vi "Cal RHS (Numeric).vi"(8 "error in (no error)":errorcluster, 10 "RHS in":variant, 11 "Domain_Steady_2D_Polygon in":refnum<class "NI_Domain_Steady_2D_Polygon.lvclass">) -> (0 "error out":errorcluster, 2 "RHS out":variant, 3 "Domain_Steady_2D_Polygon out":refnum<class "NI_Domain_Steady_2D_Polygon.lvclass">)   [LabVIEW 2017, in "NI_PDE.lvlib" / "NI_Domain_Steady_2D_Polygon.lvclass"]
uses:
  <vilib>/gmath/pde.llb/DomainClass/Domain_Steady_2D_Polygon/NI_Domain_Steady_2D_Polygon.lvclass
  <vilib>/gmath/pde.llb/DomainClass/Domain_Steady_2D_Polygon/NI_Domain_Steady_2D_Polygon.lvclass/NI_Domain_Steady_2D_Polygon.ctl
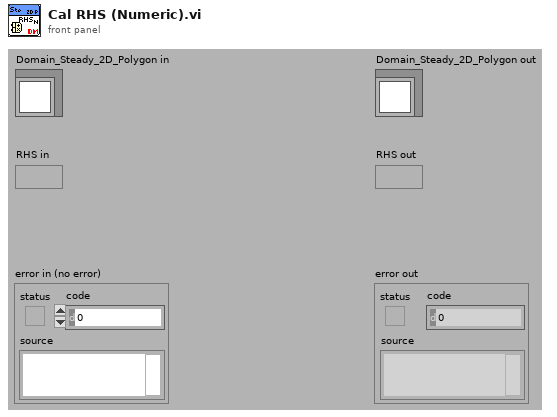
[diagram p1: front panel]
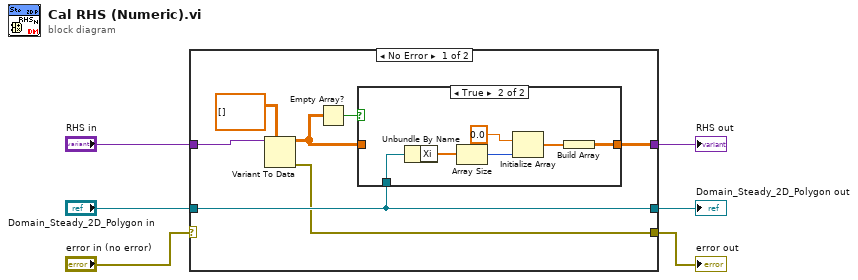
[diagram p0: block diagram]
diagram:
  n1 = case shown="No Error" "error in (no error)" {
    selector: "error in (no error)" -> [_ w23]
    tunnel: "Domain_Steady_2D_Polygon in" -> [w8 w21]
    tunnel: [w7 w23] -> w6
    tunnel: [w9 w22] -> w3
    tunnel: "RHS in" -> [w10 w22]
    tunnel: [w8 w21] -> w1
    frame No Error {
      n2 = Variant To Data(type=dbl[][] [] ("F"), Variant=w10) -> (data=w11:dbl[][], error out=w7:errorcluster)  [unwired: 1 in]
      n3 = Empty Array?(array=w11) -> (empty?=w13:bool)
      n4 = case shown="True" w13 {
        tunnel: w8 -> [_ w15]
        tunnel: w11 -> [w14 _]
        tunnel: [w14 w17] -> w9
        frame False {
        }
        frame True {
          n5 = Unbundle By Name(w15) -> ("Xi"=w16:dbl[])
          n6 = Array Size(array=w16) -> (size(s)=w20:i32)
          n7 = Initialize Array(0.0 ("element"), w20) -> (w18:dbl[])
          n8 = Build Array(w18) -> (w17:dbl[][])
        }
      }
    }
    frame Error {
    }
  }
  "Domain_Steady_2D_Polygon out" <- w1
  "error out" <- w6
  "RHS out" <- w3
